vi "test_csm_lumikki_instron_initRamp.vi"   [LabVIEW 2009]
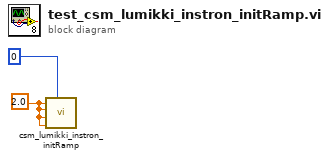
[diagram p0: block diagram]
diagram:
  w2 = 2.0 ("Set Point")
  n1 = call "csm_lumikki_instron_initRamp.vi"("ChannelInt"=0, "Ramp Rate"=w2, "Ramp Amplitude"=w2, "Set Point Time"=w2, "Set Point"=w2) -> ()  [unwired: 7 in]
